vi "Enforce Robot Rules.vi"(7 "Clust Refnum":refnum<vi>, 9 "Disable":bool, 10 "New Points":cluster{"x":dbl, "y":dbl, "th":dbl}[](array[cluster]), 11 "Original Points":cluster{"x":dbl, "y":dbl, "th":dbl}[](array[cluster])) -> (3 "Points out":cluster{"x":dbl, "y":dbl, "th":dbl}[](array[cluster]))   [LabVIEW 2020]
panel:
  # "1"
  # "2"
  # "3"
  # "4"
  # "5"
  # "6"
  # "7"
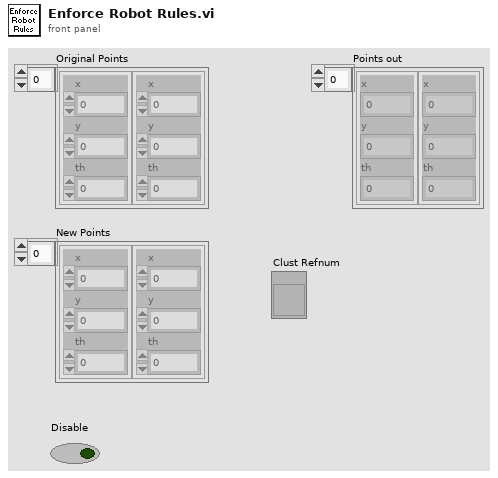
[diagram p1: front panel]
types:
  T1 = cluster{"Angular \nAccelerations":dbl[], "Override Limits?":bool[]}
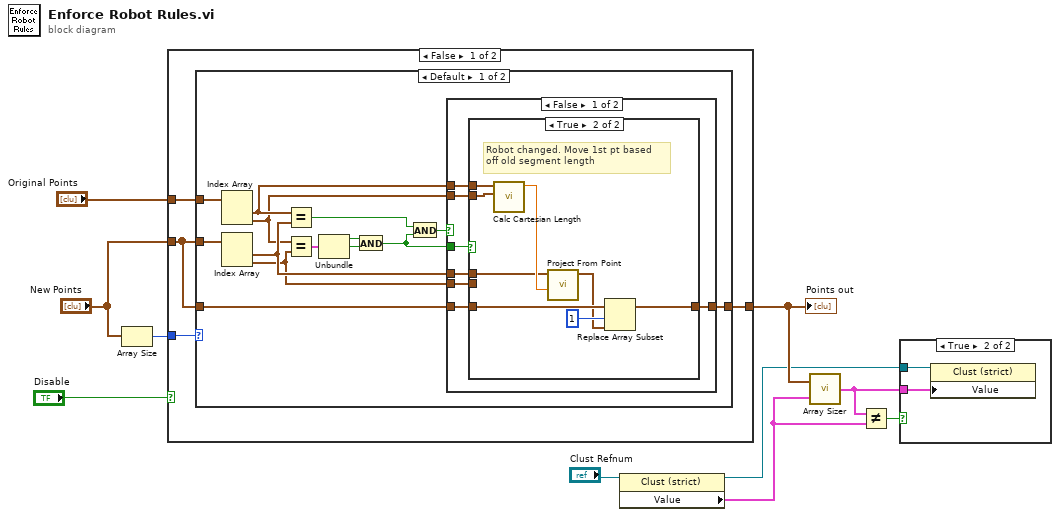
[diagram p0: block diagram]
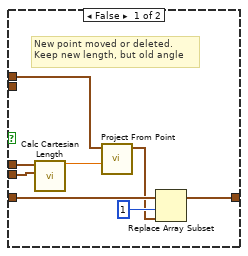
[diagram p3: hidden frame]
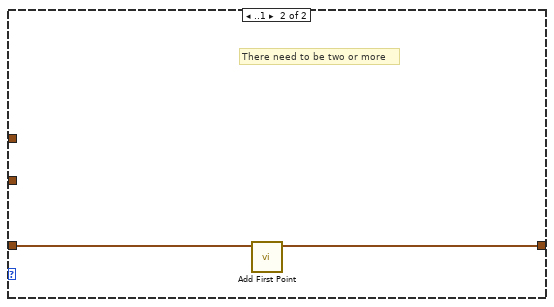
[diagram p5: hidden frame]
diagram:
  n1 = Array Size(array="New Points") -> (size(s)=w9:i32)
  n2 = case shown="False" "Disable" {
    tunnel: "Original Points" -> [w14 _]
    tunnel: w9 -> [w13 _]
    tunnel: [w12 w55] -> w6
    tunnel: "New Points" -> [w11 w55]
    frame False {
      n3 = case shown="Default" w13 {
        tunnel: w14 -> [w28 _]
        tunnel: w11 -> [w27 _]
        tunnel: [w25 w54] -> w12
        tunnel: w11 -> [w24 w53]
        frame Default {
          n4 = Index Array(array=w28) -> (element #1=w22:cluster{"x":dbl, "y":dbl, "th":dbl}, element #2=w19:cluster{"x":dbl, "y":dbl, "th":dbl})  [unwired: 2 in]
          n5 = Index Array(array=w27) -> (element #1=w21:cluster{"x":dbl, "y":dbl, "th":dbl}, element #2=w20:cluster{"x":dbl, "y":dbl, "th":dbl})  [unwired: 2 in]
          n6 = Equal?(x=w22, y=w21) -> (x = y?=w23:bool)
          n7 = Equal?(x=w19, y=w20) -> (x = y?=w18:cluster{"x":bool, "y":bool, "th":bool})
          n8 = Unbundle(w18) -> ("x"=w17:bool, "y"=w16:bool)  [unwired: 1 out]
          n9 = And(x=w17, y=w16) -> (x .and. y?=w15:bool)
          n10 = And(x=w23, y=w15) -> (x .and. y?=w26:bool)
          n11 = case shown="False" w26 {
            tunnel: [w31 w52] -> w25
            tunnel: w24 -> [w29 w52]
            tunnel: w15 -> [w33 _]
            tunnel: w22 -> [w35 _]
            tunnel: w19 -> [w34 _]
            tunnel: w21 -> [w32 _]
            tunnel: w20 -> [w30 _]
            frame False {
              n12 = case shown="True" w33 {
                tunnel: w35 -> [w38 w51]
                tunnel: w34 -> [_ w50]
                tunnel: w32 -> [w43 w45]
                tunnel: [w39 w48] -> w31
                tunnel: w30 -> [w42 _]
                tunnel: w29 -> [w40 w49]
                frame False {
                  # "New point moved or deleted.\nKeep new length, but old angle"
                  n13 = call "Calc Cartesian Length.vi"("Point 2"=w42, "Point 1"=w43) -> ("Length (f)"=w37:dbl)  [unwired: 8 in, 1 out]
                  n14 = call "Project From Point.vi"("distance"=w37, "Point In"=w38) -> ("Point Out"=w36:cluster{"x":dbl, "y":dbl, "th":dbl})  [unwired: 9 in]
                  n15 = Replace Array Subset(array=w40, new element=w36, index=1) -> (w39:cluster{"x":dbl, "y":dbl, "th":dbl}[])
                }
                frame True {
                  # "Robot changed. Move 1st pt based\noff old segment length"
                  n16 = call "Calc Cartesian Length.vi"("Point 2"=w50, "Point 1"=w51) -> ("Length (f)"=w46:dbl)  [unwired: 8 in, 1 out]
                  n17 = call "Project From Point.vi"("distance"=w46, "Point In"=w45) -> ("Point Out"=w44:cluster{"x":dbl, "y":dbl, "th":dbl})  [unwired: 9 in]
                  n18 = Replace Array Subset(array=w49, new element=w44, index=1) -> (w48:cluster{"x":dbl, "y":dbl, "th":dbl}[])
                }
              }
            }
            frame True {
              # "First two elements didn't\nchange. assume they are\ngood"
            }
          }
        }
        frame ..1 {
          # "There need to be two or more"
          n19 = call "Add First Point.vi"("Initial Points"=w53) -> ("Points"=w54:cluster{"x":dbl, "y":dbl, "th":dbl}[])  [unwired: 10 in]
        }
      }
    }
    frame True {
    }
  }
  "Points out" <- w6
  n20 = property class="Clust (strict)"(reference="Clust Refnum") -> (reference out=w4:refnum<vi>, "Value"=w2:T1)  [unwired: 1 in, 1 out]
  n21 = call "Array Sizer.vi"("Angular Accelerations"=w2, "Points out"=w6) -> ("output cluster"=w3:T1)
  n22 = Not Equal?(x=w3, y=w2) -> (x != y?=w1:bool)
  n23 = case shown="True" w1 {
    tunnel: w3 -> [_ w57]
    tunnel: w4 -> [_ w56]
    frame False {
    }
    frame True {
      n24 = property class="Clust (strict)"(reference=w56, "Value"=w57) -> ()  [unwired: 1 in, 2 out]
    }
  }
